vi "h.ACQ.SetFullSpectrumStreamToStorageAverage.vi"(8 "error in":errorcluster, 9 "Number of Averages":i32, 10 "Timeout":i32=10000, 11 "Connection ID In":refnum<k5>) -> (0 "error out":errorcluster, 3 "Connection ID Out":refnum<k5>)   [LabVIEW 2016, in "h.Library.lvlib"]
doc: "Use this vi to setup the data rate divider for streaming. (e.g., set to 10 to stream every 10th data set; set to 1 to stream every data set)\n\n<b>Connection ID In</b> - is a network connection refnum that uniquely identifies the TCP connection\n<b>Timeout</b> - specifies the maximum amount of time, in milliseconds, for the function to complete\n<b>Data Rate Divider</b> - sets the interleave for data streaming \n<b>error in</b> - describes error conditions that occur before this node runs. This input provides standard\n<b>Connection ID Out</b> - returns the same value as connection ID\n<b>error out</b> - contains error information. This output provides standard error out functionality."
uses:
  h.Library.lvlib
panel:
  # "Hyperion Set Full Spectrum\nStream to Storage Average"
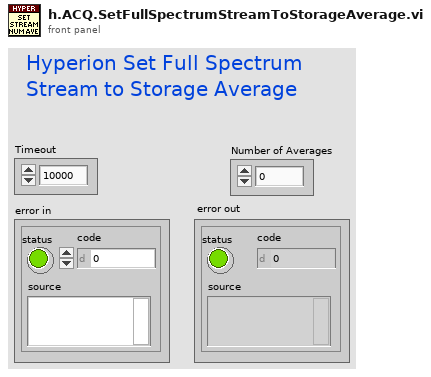
[diagram p1: front panel]
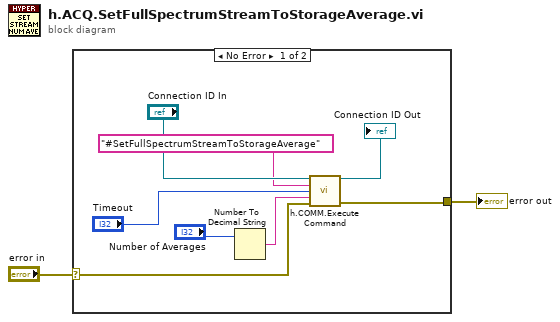
[diagram p0: block diagram]
diagram:
  n1 = case shown="No Error" "error in" {
    selector: "error in" -> [w9 w11]
    tunnel: [w8 w11] -> w1
    frame No Error {
      n2 = Number To Decimal String(number="Number of Averages") -> (decimal integer string=w3:string)  [unwired: 1 in]
      n3 = call "h.COMM.Execute Command.vi"("Connection ID"="Connection ID In", "Command"="#SetFullSpectrumStreamToStorageAverage", "Timeout"="Timeout", "Argument"=w3, "error in"=w9) -> ("Connection ID out"=→"Connection ID Out":refnum<k5>, "error out"=w8:errorcluster)  [unwired: 3 in, 6 out]
    }
    frame Error {
    }
  }
  "error out" <- w1
